vi "Calculate DNL.vi"(8 "Error In":errorcluster, 11 "DAC in":refnum<class "DAC.lvclass">) -> (0 "Error Out":errorcluster, 2 "DNL Values":dbl[](array[numeric]), 3 "DAC out":refnum<class "DAC.lvclass">)   [LabVIEW 2023, in "DAC.lvclass"]
uses:
  DAC.lvclass
  C:/Users/Ancy.Augustin/Downloads/INL DNL/INL DNL/Classes/Mode/Mode.lvclass
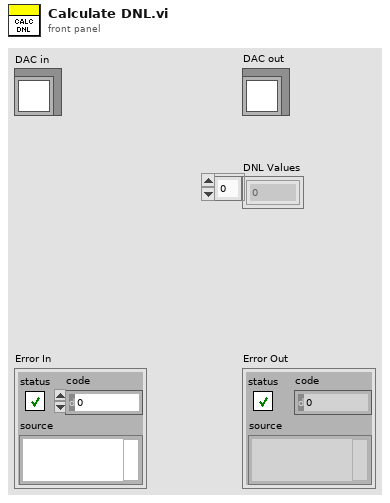
[diagram p1: front panel]
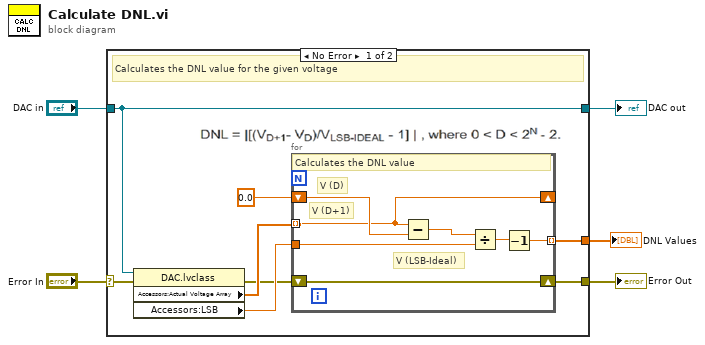
[diagram p0: block diagram]
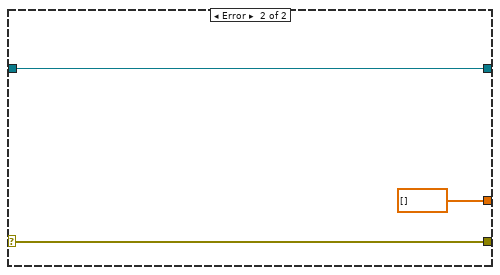
[diagram p2: hidden frame]
diagram:
  n1 = case shown="No Error" "Error In" {
    selector: "Error In" -> [w13 w23]
    tunnel: [w6 w23] -> w4
    tunnel: [w10 w22] -> w2
    tunnel: "DAC in" -> [w10 w22]
    tunnel: [w11 dbl[] []] -> w1
    frame No Error {
      # "Calculates the DNL value for the given voltage"
      n2 = property class="DAC.lvclass"(reference=w10, error in=w13) -> (error out=w7:errorcluster, "Accessors:Actual Voltage Array"=w9:dbl[], "Accessors:LSB"=w8:dbl)  [unwired: 1 out]
      n3 = for {
        tunnel: w9 -> [w15] mode=indexing
        shift-right: [w15] -> _
        shift-left: 0.0 -> [w20]
        tunnel: w8 -> [w18]
        tunnel: [w16] -> w11 mode=indexing
        shift-right: [w14] -> w6
        shift-left: w7 -> [w14]
        # "V (LSB-Ideal)"
        # "V (D+1)"
        # "V (D)"
        # "Calculates the DNL value"
        n4 = Subtract(x=w15, y=w20) -> (x-y=w19:dbl)
        n5 = Divide(x=w19, y=w18) -> (x/y=w17:dbl)
        n6 = Decrement(x=w17) -> (x-1=w16:dbl)
      }
    }
    frame Error {
    }
  }
  "Error Out" <- w4
  "DAC out" <- w2
  "DNL Values" <- w1
